vi "Test IV Plugin.vi"() -> ()   [LabVIEW 2020]
uses:
  lvsrc/Classes/Settings/Dot Settings/TypeDefs/IV Settings.ctl
  <userlib>/LevyLab/Relay Box/Type_defs/Resistor--enum.ctl
  lvsrc/Classes/Settings/Dot Settings/Dot Settings.lvclass
panel:
  in  "IV Settings":T1
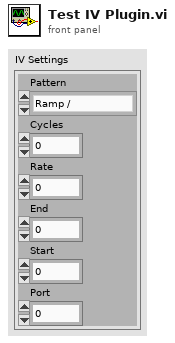
[diagram p1: front panel]
types:
  T1 = typedef "Dot Settings.lvclass/IV Settings.ctl" = cluster{"Pattern":enum16{"Ramp /", "Ramp /\\", "Smooth Ramp _/", "Smooth Ramp _/\\_", "Frequency"}, "Cycles":i32, "Rate":dbl, "End":dbl, "Start":dbl, "Port":u32}
  T2 = typedef "Resistor--enum.ctl" = enum16{"open", "discharge tip", "0 ohms", "100k ohm", "10M ohm", "1G ohm"}
  T3 = cluster{"Name":string, "Litho":cluster{"X":dbl, "Y":dbl, "Speed":dbl, "Voltage":dbl}[], "Set Resistance":T2, "Meta":variant}
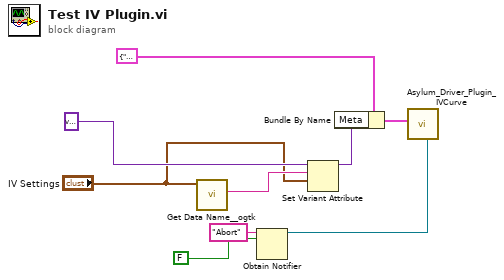
[diagram p0: block diagram]
diagram:
  n1 = call <userlib>:"Get Data Name__ogtk.vi"("Data"="IV Settings") -> ("Data Name"=w9:string)  [unwired: 8 in, 2 out]
  n2 = Obtain Notifier(name (unnamed)="Abort", notification data type=FALSE) -> (notifier out=w1:refnum<notifier>)  [unwired: 2 in, 2 out]
  n3 = Set Variant Attribute(Variant=variant, name=w9, value="IV Settings") -> (Variant out=w5:variant)  [unwired: 1 in, 2 out]
  n4 = Bundle By Name(cluster=T3 {"Name"="d0", "Litho"=[], "Set Resistance"=enum."1G ohm", "Meta"=variant} ("Pattern Data"), "Meta"=w5) -> (w4:T3)
  n5 = call "Asylum_Driver_Plugin_IVCurve.vi"("Abort Notifier"=w1, "Pattern Data"=w4) -> ()  [unwired: 6 in, 4 out]
